vi "Get and Format Time (String).vi"() -> (0 "Formatted Time":string)   [LabVIEW 2016]
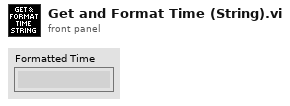
[diagram p1: front panel]
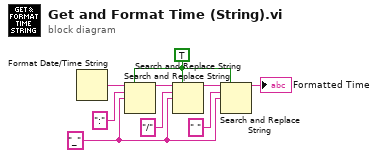
[diagram p0: block diagram]
diagram:
  w2 = "_" ("replace string (\"\")")
  w9 = TRUE ("replace all? (F)")
  n1 = Format Date/Time String() -> (date/time string=w8:string)  [unwired: 3 out]
  n2 = Search and Replace String(replace all?=w9, input string=w8, search string=":" ("substring (\"\")"), replace string=w2) -> (result string=w5:string)  [unwired: 1 in, 6 out]
  n3 = Search and Replace String(replace all?=w9, input string=w5, search string="/" ("substring (\"\")"), replace string=w2) -> (result string=w7:string)  [unwired: 1 in, 6 out]
  n4 = Search and Replace String(replace all?=w9, input string=w7, search string=" " ("substring (\"\")"), replace string=w2) -> (result string=→"Formatted Time":string)  [unwired: 1 in, 6 out]
